vi "Write I2C Slave Address (0x40).vi"(8 "error in (no error)":errorcluster, 10 "I2C Slave Address (0x40)":u8=64 format="%.0x", 11 "LINX-PCA9865 PWM in":refnum<class "LINX-PCA9685 PWM.lvclass">) -> (0 "error out":errorcluster, 3 "LINX-PCA9865 PWM out":refnum<class "LINX-PCA9685 PWM.lvclass">)   [LabVIEW 2020]
uses:
  LINX-PCA9685 PWM.lvclass
  LINX-PCA9685 PWM.lvclass/LINX-PCA9685 PWM.ctl
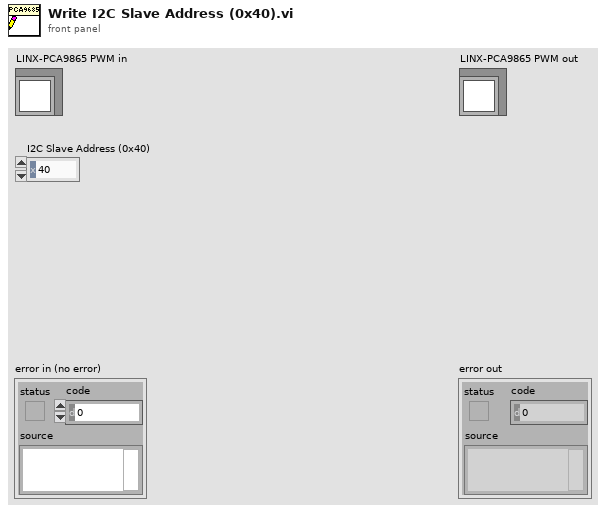
[diagram p1: front panel]
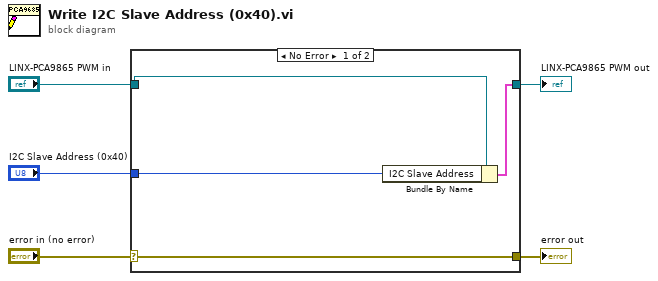
[diagram p0: block diagram]
diagram:
  n1 = case shown="No Error" "error in (no error)" {
    selector: "error in (no error)" -> [w9 w10]
    tunnel: [w9 w10] -> w4
    tunnel: [w7 w11] -> w2
    tunnel: "LINX-PCA9865 PWM in" -> [w8 w11]
    tunnel: "I2C Slave Address (0x40)" -> [w6 _]
    frame No Error {
      n2 = Bundle By Name(cluster=w8, "I2C Slave Address"=w6) -> (w7:cluster{})
    }
    frame Error {
    }
  }
  "error out" <- w4
  "LINX-PCA9865 PWM out" <- w2
